vi "Init.vi"(8 "error in (no error)":errorcluster caption="Error in", 11 "Com in":refnum<visa-resource-name>="COM1") -> (0 "Error out":errorcluster, 3 "Com out":refnum<visa-resource-name>)   [LabVIEW 2020]
uses:
  <vilib>/Instr/_visa.llb/VISA Configure Serial Port (Instr).vi
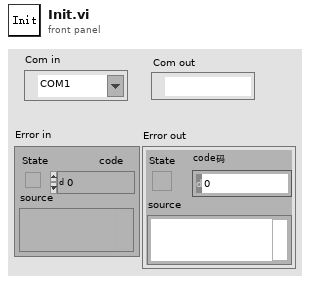
[diagram p1: front panel]
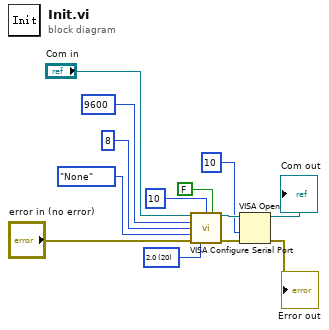
[diagram p0: block diagram]
diagram:
  w7 = u16 20 items=["1.0"=10, "1.5"=15, "2.0"=20] ("stop bits (10: 1 bit)")
  n1 = call-poly "VISA Configure Serial Port"("VISA resource name"="Com in", "termination char\n(0xA = '\\n' = LF)"=u8 10 ("termination char\n(0xA = '\\n' = LF)"), "Enable Termination\nChar (T)"=FALSE ("Enable Termination\nChar (T)"), "baud rate (9600)"=u32 9600 ("波特率"), "data bits (8)"=u16 8 ("bits (8)"), "parity (0:none)"=enum16{"None", "Odd", "Even", "Mark", "Space"}."None", "error in (no error)"="error in (no error)", "stop bits (10: 1 bit)"=w7) -> ("VISA resource name out"=w11:refnum<visa-resource-name>, "error out"=w9:errorcluster)  [unwired: 6 in]
  n2 = VISA Open(access mode=u32 10, error in (no error)=w9, VISA resource name=w11) -> (VISA resource name=→"Com out":refnum<visa-resource-name>, error out=→"Error out":errorcluster)  [unwired: 2 in]
